vi "SS2 Live_Update Gate Definition.vi"(8 "error in (no error)":errorcluster, 10 "Gate Configuration Definition":T1, 11 "SS2 DAQ Parameters Refnum":refnum<vi>) -> (0 "error out":errorcluster, 2 "SS2 DAQ Parameters":T3 {"Sync Period" min=0.0 max=4.294967295; "# Sets" min=1})   [LabVIEW 2019]
uses:
  SS2 DAQ Parameters 3.ctl
  SS2 Gate Definition.ctl
  SS2 Gate Configuration.ctl
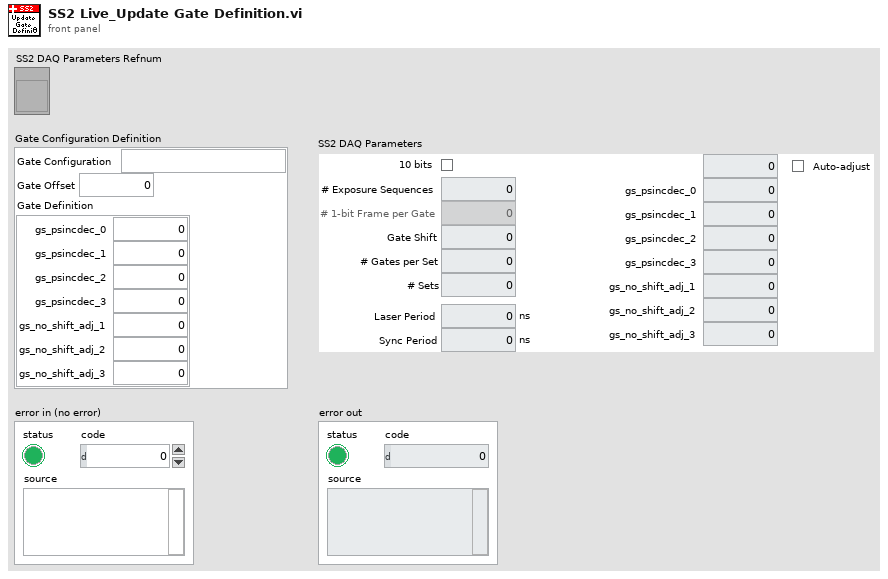
[diagram p1: front panel]
types:
  T1 = typedef "SS2 Gate Configuration.ctl" = cluster{"Gate Configuration":string, "Gate Offset":u32, "Gate Definition":T2}
  T2 = typedef "SS2 Gate Definition.ctl" = cluster{"gs_psincdec_0":u32, "gs_psincdec_1":u32, "gs_psincdec_2":u32, "gs_psincdec_3":u32, "gs_no_shift_adj_1":u32, "gs_no_shift_adj_2":u32, "gs_no_shift_adj_3":u32}
  T3 = typedef "SS2 DAQ Parameters 3.ctl" = cluster{"10 bits":bool, "# Exposure Sequences":u32, "# 1-bit Frame per Gate":u32, "Gate Shift":u32, "# Gates per Set":u32, "# Sets":u32, "Laser Period":dbl[unit], "Sync Period":dbl[unit], "Gate Offset":u32, "Auto-adjust Gate Offset":bool, "Gate Definition":T2}
  T4 = typedef "SS2 DAQ Parameters 2.ctl" = cluster{"10 bits":bool, "# Exposure Sequences":u32, "# 1-bit Frame per Gate":u32, "Gate Shift":u32, "# Gates per Set":u32, "# Sets":u32, "Laser Period":dbl[unit], "Sync Period":dbl[unit], "Gate Offset":u32, "Auto-adjust Gate Offset":bool, "Gate Definition":T2}
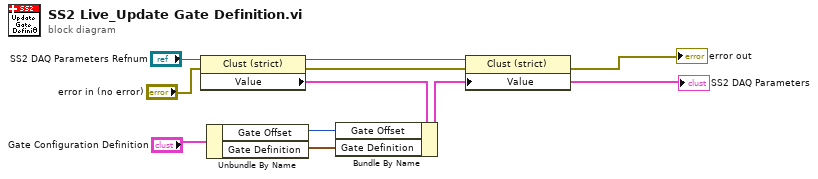
[diagram p0: block diagram]
diagram:
  n1 = property class="Clust (strict)"(reference="SS2 DAQ Parameters Refnum", error in="error in (no error)") -> (reference out=w9:refnum<vi>, error out=w8:errorcluster, "Value"=w5:T4)
  n2 = Unbundle By Name("Gate Configuration Definition") -> ("Gate Offset"=w3:u32, "Gate Definition"=w2:T2)
  n3 = Bundle By Name(cluster=w5, "Gate Offset"=w3, "Gate Definition"=w2) -> (w4:T4)
  "SS2 DAQ Parameters" <- w4
  n4 = property class="Clust (strict)"(reference=w9, error in=w8, "Value"=w4) -> (error out=→"error out":errorcluster)  [unwired: 1 out]
